vi "Battery Life Calculator.vi"(1 "Battery Size (Ah)":dbl, 2 "Amps":dbl) -> (0 "Battery Life (h)":dbl)   [LabVIEW 2014]
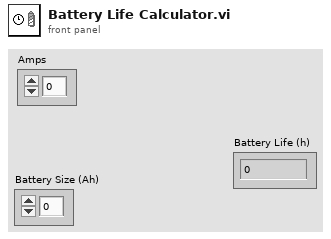
[diagram p1: front panel]
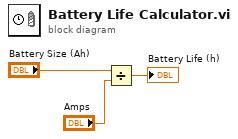
[diagram p0: block diagram]
diagram:
  n1 = Divide(x="Battery Size (Ah)", y="Amps") -> (x/y=→"Battery Life (h)":dbl)
